vi "Autonomous Independent.vi"   [LabVIEW 2019]
doc: "This VI is called when autonomous begins, and will automatically be terminated when autonomous ends. You can carry out timed or sensor driven robot movement independently without needing to return to the caller."
uses:
  <vilib>/Rock Robotics/WPI/Solenoid/WPI_SolenoidValue.ctl
  <vilib>/Rock Robotics/WPI/ThirdParty/Phoenix-LabVIEW/Motor Controller/Controls/CTRE_Phoenix_MotorControl_ControlMode.ctl
  <vilib>/Rock Robotics/WPI/Utilities/WPI_GetSetVariantRefNum.vi
  <vilib>/Rock Robotics/Network Tables/NT Read String.vi
  <vilib>/Rock Robotics/Network Tables/NT Write Numeric Array.vi
  <vilib>/Rock Robotics/WPI/Solenoid/WPI_SolenoidSetEnum.vi
  <vilib>/addons/control/pid/pid.llb/PID (DBL).vi
  <vilib>/Rock Robotics/Network Tables/NT Read Number.vi
  <vilib>/Rock Robotics/WPI/RobotDrive/WPI_RobotDriveArcadeDrive_Standard(NoSaturation).vi
  <vilib>/Rock Robotics/Network Tables/NT Write Number.vi
  <vilib>/addons/control/pid/NI_PID_pid.lvlib
panel:
  # "Be sure to right-click and choose Data Operations>>Make Current Value default if you want to save the array values with the VI"
types:
  T1 = typedef "WPI_JoystickDevRef.ctl" = cluster{"Device":T2}
  T2 = typedef "WPI_JoystickDeviceEnum.ctl" = enum16{"USB 0", "USB 1", "USB 2", "USB 3", "USB 4", "USB 5"}
  T3 = typedef "WPI_SolenoidValue.ctl" = enum16{"Off", "On", "Forward", "Reverse"}
  T4 = cluster{"proportional gain (Kc)":dbl, "integral time (Ti, min)":dbl, "derivative time (Td, min)":dbl}
  T5 = typedef "WPI_SolenoidDevRef.ctl" = cluster{"DevStatus":errorcluster, "Pneumatics Control Module":u8, "Forward Solenoid Channel":T6, "Reverse Solenoid Channel":T6}
  T6 = typedef "WPI_SolenoidChannel.ctl" = enum8{"Solenoid 0", "Solenoid 1", "Solenoid 2", "Solenoid 3", "Solenoid 4", "Solenoid 5", "Solenoid 6", "Solenoid 7", "Invalid"}
  T7 = typedef "CTRE_Phoenix_MotorControl_ControlMode.ctl" = u16
  T8 = typedef "WPI_SwitchDevRef.ctl" = cluster{"DevStatus":errorcluster, "DIO Channel":T9, "CntIndex":T10, "Normally Closed":bool}
  T9 = typedef "FPGA_DIOChannel.ctl" = enum8{"DIO 0", "DIO 1", "DIO 2", "DIO 3", "DIO 4", "DIO 5", "DIO 6", "DIO 7", "DIO 8", "DIO 9", "DIO MXP 0", "DIO MXP 1", "DIO MXP 2", "DIO MXP 3", "DIO MXP 4", "DIO MXP 5", "DIO MXP 6", "DIO MXP 7", "DIO MXP 8", "DIO MXP 9", "DIO MXP 10", "DIO MXP 11", "DIO MXP 12", "DIO MXP 13", "DIO MXP 14", "DIO MXP 15", "SPI Port CS1", "SPI Port CS2", "SPI Port CS3", "SPI Port MISO", "SPI Port MOSI", "Invalid"}
  T10 = typedef "FPGA_CounterCtrSystemIndex.ctl" = enum8{"Ctr 0", "Ctr 1", "Ctr 2", "Ctr 3", "Ctr 4", "Ctr 5", "Ctr 6", "Ctr 7", "Invalid"}
  T11 = typedef "WPI_MotorControlDeviceRef.ctl" = cluster{"DeviceStatus":errorcluster, "Type":T12, "PWM":cluster{"PWM Channel":T13, "DeadBand":T14}, "CAN":cluster{"Device Number":u8, "SetOutput VI Ref":variant, "GetOutput VI Ref":variant, "Enable VI Ref":variant, "Disable VI Ref":variant, "Data":variant}, "Invert":bool, "DIO PWM":cluster{"PWM \"Enable\" Channel":T13, "DIOChannel":T9, "PWM Rate":dbl}}
  T12 = typedef "WPI_MotorControlType.ctl" = enum16{"PWM", "CAN", "DIO PWM"}
  T13 = typedef "FPGA_DIOPWMChannel.ctl" = enum8{"PWM 0", "PWM 1", "PWM 2", "PWM 3", "PWM 4", "PWM 5", "PWM 6", "PWM 7", "PWM 8", "PWM 9", "PWM MXP 0", "PWM MXP 1", "PWM MXP 2", "PWM MXP 3", "PWM MXP 4", "PWM MXP 5", "PWM MXP 6", "PWM MXP 7", "PWM MXP 8", "PWM MXP 9", "Invalid"}
  T14 = typedef "WPI_PWMDeadband.ctl" = cluster{"Name":string, "maxPositivePwm":i32, "minPositivePwm":i32, "centerPwm":i32, "maxNegativePwm":i32, "minNegativePwm":i32, "angularRange":u16}
  T15 = typedef "WPI_EncoderDevRef.ctl" = cluster{"DevStatus":errorcluster, "EncoderIndex":T16, "CounterIndex":T10, "DistancePerCount":dbl, "Decoding Type":T17}
  T16 = typedef "FPGA_EncoderIdx.ctl" = enum8{"Enc 0", "Enc 1", "Enc 2", "Enc 3", "Enc 4", "Enc 5", "Enc 6", "Enc 7", "Invalid"}
  T17 = typedef "WPI_EncoderType.ctl" = enum16{"1x", "2x", "4x"}
  T18 = typedef "WPI_RobotDriveDevRef.ctl" = cluster{"DevStatus":errorcluster, "Motors[]":T11[], "Square Inputs":bool, "Max Output":dbl}
  T19 = typedef "WPI_DigitalInputDevRef.ctl" = cluster{"DevStatus":errorcluster, "DIO Channel":T9}
diagram:
  (unwired) "This function is run in parallel when the autonomous period begins. It will be terminated automatically when the period ends.\n\nNote that all Driver Station inputs are automatically latched and will not change once auto begins."
  # "The game specific data sent by FMS"
  # "This tells you the autonomous selected in the \ndashboard. Begin.vi publishes the Auto List values\nby writing a constant to the dashboard.\nUpdate the constant to add or modify the name\nof an autonomous."
  # "Every 20ms, report that we are running autonomous\ncode. Loop will abort the same time as the VI."
  # "This gives you the joystick value\nthat is often the throttle"
  # "Use time and/or sensors to control how the robot drives."
  # "This tells you the driver position\nand alliance color"
  n1 = call <vilib>:"WPI_DriverStationGet Alliance Info.vi"() -> ()  [unwired: 12 out]
  n2 = while {
    stop <- FALSE stop-if-true
    n3 = call <vilib>:"WPI_DriverStationReport Robot Code State.vi"("Autonomous"=TRUE) -> ()  [unwired: 10 in, 1 out]
    n4 = Wait (ms)(milliseconds to wait=u32 20) -> ()  [unwired: 1 out]
  }
  n5 = call <vilib>:"WPI_JoystickRefNum Registry Get.vi"("refnum name"="Joystick 0") -> ("JoystickDevRef"=w7:T1)  [unwired: 1 in, 9 out]
  n6 = call <vilib>:"WPI_JoystickGetValues.vi"("JoystickDevRef"=w7) -> ("Axes"=w3:dbl[])  [unwired: 6 in, 4 out]
  n7 = Index Array(array=w3, index=2) -> ()  [unwired: 1 out]
  n8 = call-poly <vilib>:"NT Write Value.vi"("Numeric Array"=w3, "Name"="Joystick 0/Axes") -> ()  [unwired: 9 in, 1 out]
  n9 = call <vilib>:"WPI_DriverStationGame Specific Data.vi"() -> ("Game Specific Data"=w1:string)  [unwired: 11 in]
  n10 = call-poly <vilib>:"NT Read Value.vi"("Name"="Auto Selector") -> ("String"=w4:string)  [unwired: 9 in, 1 out]
  n11 = case shown="\"a\"" w4 {
    tunnel: w1 -> [_ _ _ _ _ _]
    frame Default {
    }
    frame "acc" {
    }
    frame "a" {
      n12 = flat-sequence {
        tunnel: [w67] -> w14
        tunnel: [w66] -> w13
        tunnel: w14 -> [w88]
        tunnel: w13 -> [w89]
        tunnel: [w121] -> w12
        tunnel: w12 -> [w149]
        frame #0 {
          # "turn the light"
          n13 = call <vilib>:"WPI_SolenoidRefNum Registry Get.vi"("refnum name"="led") -> ("error out"=w18:errorcluster, "SolenoidDevRef"=w17:T5)  [unwired: 9 in]
          n14 = call-poly <vilib>:"WPI_SolenoidSet.vi"("error in (no error)"=w18, "Value"=WPI_SolenoidValue."On", "SolenoidDevRef"=w17) -> ()  [unwired: 7 in, 2 out]
        }
        frame #1 {
          w26 = T7 0 items=["PercentOutput"=0, "Position"=1, "Velocity"=2, "Current"=3, "Follower"=5, "MotionProfile"=6, "MotionMagic"=7, "MotionProfileArc"=10, "Disabled"=15] ("Control Mode")
          # "reset all the encoder"
          n15 = while {
            tunnel: [w31] -> w25
            tunnel: [w30] -> w23
            stop <- w30 stop-if-true
            w36 = T7 0 items=["PercentOutput"=0, "Position"=1, "Velocity"=2, "Current"=3, "Follower"=5, "MotionProfile"=6, "MotionMagic"=7, "MotionProfileArc"=10, "Disabled"=15] ("Control Mode")
            n16 = call <vilib>:"WPI_SwitchRefNum Registry Get.vi"("refnum name"="stop") -> ("error out"=w41:errorcluster, "SwitchDevRef"=w40:T8)  [unwired: 9 in]
            n17 = case shown="True" TRUE {
              frame False {
              }
              frame True {
                n18 = call <vilib>:"Zero Yaw.vi"("Zero"=TRUE) -> ()  [unwired: 11 in]
              }
            }
            n19 = call <vilib>:"WPI_SwitchGetLimitValue.vi"("error in (no error)"=w41, "SwitchDevRef"=w40) -> ("Switch Pressed"=w33:bool)  [unwired: 7 in, 2 out]
            n20 = call <vilib>:"CTRE_Phoenix_MotorControl_RefNumRegistryGet.vi"("refnum name"="chain") -> ("error out"=w38:errorcluster, "PhoenixMotorControlDevRef"=w37:T11)  [unwired: 9 in]
            n21 = Equal?(x=w33, y=TRUE) -> (x = y?=w30:bool)
            n22 = call <vilib>:"CTRE_Phoenix_MotorControl_Set.vi"("error in (no error)"=w38, "Output"=-0.8, "Control Mode"=w36, "PhoenixMotorControlDevRef"=w37) -> ("PhoenixMotorControlDevRef"=w31:T11)  [unwired: 6 in, 1 out]
          }
          n23 = call <vilib>:"WPI_EncoderRefNum Registry Get.vi"("refnum name"="angle") -> ("EncoderDevRef"=w19:T15)  [unwired: 9 in, 1 out]
          n24 = call <vilib>:"WPI_EncoderRefNum Registry Get.vi"("refnum name"="move") -> ("EncoderDevRef"=w20:T15)  [unwired: 9 in, 1 out]
          n25 = case shown="True" w23 {
            tunnel: w20 -> [_ w28]
            tunnel: w19 -> [_ w27]
            frame False {
            }
            frame True {
              n26 = call <vilib>:"WPI_EncoderReset.vi"("EncoderDevRef"=w27) -> ()  [unwired: 9 in, 2 out]
              n27 = call <vilib>:"WPI_EncoderReset.vi"("EncoderDevRef"=w28) -> ()  [unwired: 9 in, 2 out]
            }
          }
          n28 = call <vilib>:"CTRE_Phoenix_MotorControl_Set.vi"("Output"=0.0, "Control Mode"=w26, "PhoenixMotorControlDevRef"=w25) -> ()  [unwired: 7 in, 2 out]
        }
        frame #2 {
          w44 = T7 0 items=["PercentOutput"=0, "Position"=1, "Velocity"=2, "Current"=3, "Follower"=5, "MotionProfile"=6, "MotionMagic"=7, "MotionProfileArc"=10, "Disabled"=15] ("Control Mode")
          # "set angle"
          n29 = while {
            tunnel: [w46] -> w45
            stop <- w50 stop-if-true
            w48 = -323.0 ("setpoint")
            w47 = T7 0 items=["PercentOutput"=0, "Position"=1, "Velocity"=2, "Current"=3, "Follower"=5, "MotionProfile"=6, "MotionMagic"=7, "MotionProfileArc"=10, "Disabled"=15] ("Control Mode")
            n30 = call <vilib>:"WPI_EncoderRefNum Registry Get.vi"("refnum name"="angle") -> ("error out"=w57:errorcluster, "EncoderDevRef"=w58:T15)  [unwired: 9 in]
            n31 = call <vilib>:"WPI_EncoderGet.vi"("error in (no error)"=w57, "EncoderDevRef"=w58) -> ("Distance"=w49:dbl)  [unwired: 4 in, 5 out]
            n32 = call-poly <vilib>:"PID.vi"("output range"=cluster{"output high":dbl, "output low":dbl} {"output high"=0.8, "output low"=-0.8}, "PID gains"=T4 {"proportional gain (Kc)"=0.02, "integral time (Ti, min)"=0.0, "derivative time (Td, min)"=0.0}, "process variable"=w49, "setpoint"=w48) -> ("output"=w60:dbl)  [unwired: 6 in, 1 out]
            n33 = call <vilib>:"CTRE_Phoenix_MotorControl_RefNumRegistryGet.vi"("refnum name"="chain") -> ("error out"=w63:errorcluster, "PhoenixMotorControlDevRef"=w64:T11)  [unwired: 9 in]
            n34 = Multiply(x=w60, y=-1.0) -> (x*y=w55:dbl)
            n35 = Add(x=w48, y=-2.0) -> (x+y=w51:dbl)
            n36 = Add(x=w48, y=2.0) -> (x+y=w53:dbl)
            n37 = call <vilib>:"CTRE_Phoenix_MotorControl_Set.vi"("error in (no error)"=w63, "Output"=w55, "Control Mode"=w47, "PhoenixMotorControlDevRef"=w64) -> ("PhoenixMotorControlDevRef"=w46:T11)  [unwired: 6 in, 1 out]
            n38 = In Range and Coerce(upper limit=w53, x=w49, lower limit=w51) -> (In Range?=w50:bool)  [unwired: 1 out]
          }
          n39 = call <vilib>:"CTRE_Phoenix_MotorControl_Set.vi"("Output"=0.0, "Control Mode"=w44, "PhoenixMotorControlDevRef"=w45) -> ()  [unwired: 7 in, 2 out]
        }
        frame #3 {
          # "get the wheel shoot"
          # "preparation"
          n40 = Tick Count (ms)() -> (millisecond timer value=w68:u32)
          n41 = while {
            tunnel: w68 -> [w74]
            tunnel: [w70] -> w66
            tunnel: [w69] -> w67
            stop <- w71 stop-if-true
            w80 = T7 0 items=["PercentOutput"=0, "Position"=1, "Velocity"=2, "Current"=3, "Follower"=5, "MotionProfile"=6, "MotionMagic"=7, "MotionProfileArc"=10, "Disabled"=15] ("Control Mode")
            w84 = T7 0 items=["PercentOutput"=0, "Position"=1, "Velocity"=2, "Current"=3, "Follower"=5, "MotionProfile"=6, "MotionMagic"=7, "MotionProfileArc"=10, "Disabled"=15] ("Control Mode")
            n42 = Tick Count (ms)() -> (millisecond timer value=w75:u32)
            n43 = Subtract(x=w75, y=w74) -> (x-y=w73:u32)
            n44 = call <vilib>:"CTRE_Phoenix_MotorControl_RefNumRegistryGet.vi"("refnum name"="shoot1") -> ("PhoenixMotorControlDevRef"=w78:T11)  [unwired: 9 in, 1 out]
            n45 = Greater Or Equal?(x=w73, y=u32 3000) -> (x >= y?=w71:bool)
            n46 = call <vilib>:"CTRE_Phoenix_MotorControl_RefNumRegistryGet.vi"("refnum name"="shoot2") -> ("error out"=w82:errorcluster, "PhoenixMotorControlDevRef"=w83:T11)  [unwired: 9 in]
            n47 = call <vilib>:"CTRE_Phoenix_MotorControl_Set.vi"("Output"=-1.0, "Control Mode"=w80, "PhoenixMotorControlDevRef"=w78) -> ("PhoenixMotorControlDevRef"=w69:T11)  [unwired: 7 in, 1 out]
            n48 = call <vilib>:"CTRE_Phoenix_MotorControl_Set.vi"("error in (no error)"=w82, "Output"=1.0, "Control Mode"=w84, "PhoenixMotorControlDevRef"=w83) -> ("PhoenixMotorControlDevRef"=w70:T11)  [unwired: 6 in, 1 out]
          }
        }
        frame #4 {
          w87 = T7 0 items=["PercentOutput"=0, "Position"=1, "Velocity"=2, "Current"=3, "Follower"=5, "MotionProfile"=6, "MotionMagic"=7, "MotionProfileArc"=10, "Disabled"=15] ("Control Mode")
          w90 = T7 0 items=["PercentOutput"=0, "Position"=1, "Velocity"=2, "Current"=3, "Follower"=5, "MotionProfile"=6, "MotionMagic"=7, "MotionProfileArc"=10, "Disabled"=15] ("Control Mode")
          # "finish shooting"
          n49 = Tick Count (ms)() -> (millisecond timer value=w93:u32)
          n50 = while {
            tunnel: w93 -> [w111]
            tunnel: w88 -> [w98]
            tunnel: w89 -> [w97]
            tunnel: [w96] -> w91
            tunnel: [w95] -> w85
            tunnel: [w94] -> _
            stop <- w108 stop-if-true
            w103 = T7 0 items=["PercentOutput"=0, "Position"=1, "Velocity"=2, "Current"=3, "Follower"=5, "MotionProfile"=6, "MotionMagic"=7, "MotionProfileArc"=10, "Disabled"=15] ("Control Mode")
            w107 = T7 0 items=["PercentOutput"=0, "Position"=1, "Velocity"=2, "Current"=3, "Follower"=5, "MotionProfile"=6, "MotionMagic"=7, "MotionProfileArc"=10, "Disabled"=15] ("Control Mode")
            w115 = T7 0 items=["PercentOutput"=0, "Position"=1, "Velocity"=2, "Current"=3, "Follower"=5, "MotionProfile"=6, "MotionMagic"=7, "MotionProfileArc"=10, "Disabled"=15] ("Control Mode")
            w116 = T7 0 items=["PercentOutput"=0, "Position"=1, "Velocity"=2, "Current"=3, "Follower"=5, "MotionProfile"=6, "MotionMagic"=7, "MotionProfileArc"=10, "Disabled"=15] ("Control Mode")
            n51 = Tick Count (ms)() -> (millisecond timer value=w112:u32)
            n52 = Subtract(x=w112, y=w111) -> (x-y=w110:u32)
            n53 = call <vilib>:"CTRE_Phoenix_MotorControl_RefNumRegistryGet.vi"("refnum name"="convey2") -> ("PhoenixMotorControlDevRef"=w101:T11)  [unwired: 9 in, 1 out]
            n54 = call <vilib>:"CTRE_Phoenix_MotorControl_RefNumRegistryGet.vi"("refnum name"="convey1") -> ("error out"=w105:errorcluster, "PhoenixMotorControlDevRef"=w106:T11)  [unwired: 9 in]
            n55 = Greater Or Equal?(x=w110, y=u32 3000) -> (x >= y?=w108:bool)
            n56 = call <vilib>:"CTRE_Phoenix_MotorControl_Set.vi"("error in (no error)"=w105, "Output"=0.5, "Control Mode"=w107, "PhoenixMotorControlDevRef"=w106) -> ("PhoenixMotorControlDevRef"=w94:T11)  [unwired: 6 in, 1 out]
            n57 = call <vilib>:"CTRE_Phoenix_MotorControl_Set.vi"("Output"=1.0, "Control Mode"=w116, "PhoenixMotorControlDevRef"=w97) -> ("PhoenixMotorControlDevRef"=w96:T11)  [unwired: 7 in, 1 out]
            n58 = call <vilib>:"CTRE_Phoenix_MotorControl_Set.vi"("Output"=-1.0, "Control Mode"=w115, "PhoenixMotorControlDevRef"=w98) -> ("PhoenixMotorControlDevRef"=w95:T11)  [unwired: 7 in, 1 out]
            n59 = call <vilib>:"CTRE_Phoenix_MotorControl_Set.vi"("Output"=0.5, "Control Mode"=w103, "PhoenixMotorControlDevRef"=w101) -> ()  [unwired: 7 in, 2 out]
          }
          n60 = call <vilib>:"CTRE_Phoenix_MotorControl_Set.vi"("Output"=0.0, "Control Mode"=w90, "PhoenixMotorControlDevRef"=w91) -> ()  [unwired: 7 in, 2 out]
          n61 = call <vilib>:"CTRE_Phoenix_MotorControl_Set.vi"("Output"=0.0, "Control Mode"=w87, "PhoenixMotorControlDevRef"=w85) -> ()  [unwired: 7 in, 2 out]
        }
        frame #5 {
          # "turn the light off"
          n62 = call <vilib>:"WPI_SolenoidRefNum Registry Get.vi"("refnum name"="led") -> ("error out"=w120:errorcluster, "SolenoidDevRef"=w119:T5)  [unwired: 9 in]
          n63 = call-poly <vilib>:"WPI_SolenoidSet.vi"("error in (no error)"=w120, "Value"=WPI_SolenoidValue."Off", "SolenoidDevRef"=w119) -> ()  [unwired: 7 in, 2 out]
        }
        frame #6 {
          # "turn 30 deg"
          n64 = Tick Count (ms)() -> (millisecond timer value=w122:u32)
          n65 = while {
            tunnel: [w129] -> w121
            tunnel: w122 -> [w126]
            stop <- w123 stop-if-true
            n66 = call-poly <vilib>:"NT Read Value.vi"("Name"="/vision/fuseheading") -> ("Numeric"=w142:dbl)  [unwired: 9 in, 1 out]
            n67 = Subtract(x=w142, y=30.0) -> (x-y=w135:dbl)
            n68 = call <vilib>:"WPI_RobotDriveRefNum Registry Get.vi"("refnum name"="Left and Right Motors") -> ("RobotDriveDevRef"=w146:T18)  [unwired: 9 in, 1 out]
            n69 = Less?(x=w135, y=-180.0 ("x-y")) -> (x < y?=w133:bool)
            n70 = Add(x=w135, y=360.0) -> (x+y=w132:dbl)
            n71 = Select(t=w132, s=w133, f=w135) -> (s? t:f=w131:dbl)
            n72 = Greater Or Equal?(x=w135, y=180.0) -> (x >= y?=w140:bool)
            n73 = Subtract(x=w135, y=360.0) -> (x-y=w139:dbl)
            n74 = Select(t=w139, s=w140, f=w131) -> (s? t:f=w128:dbl)
            n75 = Tick Count (ms)() -> (millisecond timer value=w127:u32)
            n76 = Subtract(x=w127, y=w126) -> (x-y=w125:u32)
            n77 = call-poly <vilib>:"PID.vi"("output range"=cluster{"output high":dbl, "output low":dbl} {"output high"=0.6, "output low"=-0.6}, "PID gains"=T4 {"proportional gain (Kc)"=0.13, "integral time (Ti, min)"=0.0, "derivative time (Td, min)"=0.0}, "process variable"=w128, "setpoint"=0.0) -> ("output"=w130:dbl)  [unwired: 6 in, 1 out]
            n78 = Greater Or Equal?(x=w125, y=u32 3000) -> (x >= y?=w123:bool)
            n79 = call-poly <vilib>:"WPI_RobotDriveArcadeDrive.vi"("X axis value"=w130, "RobotDriveDevRef"=w146) -> ("RobotDriveDevRef"=w129:T18)  [unwired: 7 in, 2 out]
          }
        }
        frame #7 {
          n80 = Tick Count (ms)() -> (millisecond timer value=w150:u32)
          n81 = while {
            tunnel: w150 -> [w154]
            tunnel: w149 -> [w152]
            stop <- w153 stop-if-true
            n82 = Tick Count (ms)() -> (millisecond timer value=w155:u32)
            n83 = Subtract(x=w155, y=w154) -> (x-y=w156:u32)
            n84 = Greater Or Equal?(x=w156, y=u32 2000) -> (x >= y?=w153:bool)
            n85 = call-poly <vilib>:"WPI_RobotDriveArcadeDrive.vi"("Y axis value"=0.5, "RobotDriveDevRef"=w152) -> ()  [unwired: 7 in, 3 out]
          }
        }
      }
    }
    frame "b" {
      n86 = flat-sequence {
        tunnel: [w227] -> w174
        tunnel: [w226] -> w173
        tunnel: w174 -> [w250]
        tunnel: w173 -> [w251]
        tunnel: [w249] -> w163
        tunnel: [w248] -> w161
        tunnel: w163 -> [w285]
        tunnel: [w285] -> w162
        tunnel: w161 -> [w284]
        tunnel: [w284] -> w160
        tunnel: [w287] -> w172
        tunnel: [w286] -> w171
        tunnel: [w289] -> w170
        tunnel: w162 -> [w287]
        tunnel: w160 -> [w286]
        tunnel: w172 -> [w327]
        tunnel: w171 -> [w326]
        tunnel: w170 -> [w325]
        tunnel: [w318] -> w169
        tunnel: [w317] -> w168
        tunnel: [w316] -> w167
        tunnel: w169 -> [w386]
        tunnel: [w386] -> w164
        tunnel: w168 -> [w383]
        tunnel: w167 -> [w384]
        tunnel: w164 -> [w400]
        tunnel: [w399] -> w159
        tunnel: w159 -> [w435]
        tunnel: [w435] -> w158
        tunnel: w158 -> [w438]
        tunnel: [w437] -> w166
        tunnel: [w436] -> w165
        tunnel: w166 -> [w475]
        tunnel: w165 -> [w474]
        frame #0 {
          # "turn the light"
          n87 = call <vilib>:"WPI_SolenoidRefNum Registry Get.vi"("refnum name"="led") -> ("error out"=w178:errorcluster, "SolenoidDevRef"=w177:T5)  [unwired: 9 in]
          n88 = call-poly <vilib>:"WPI_SolenoidSet.vi"("error in (no error)"=w178, "Value"=WPI_SolenoidValue."On", "SolenoidDevRef"=w177) -> ()  [unwired: 7 in, 2 out]
        }
        frame #1 {
          w186 = T7 0 items=["PercentOutput"=0, "Position"=1, "Velocity"=2, "Current"=3, "Follower"=5, "MotionProfile"=6, "MotionMagic"=7, "MotionProfileArc"=10, "Disabled"=15] ("Control Mode")
          # "reset all the encoder"
          n89 = while {
            tunnel: [w191] -> w185
            tunnel: [w190] -> w183
            stop <- w190 stop-if-true
            w196 = T7 0 items=["PercentOutput"=0, "Position"=1, "Velocity"=2, "Current"=3, "Follower"=5, "MotionProfile"=6, "MotionMagic"=7, "MotionProfileArc"=10, "Disabled"=15] ("Control Mode")
            n90 = call <vilib>:"WPI_SwitchRefNum Registry Get.vi"("refnum name"="stop") -> ("error out"=w201:errorcluster, "SwitchDevRef"=w200:T8)  [unwired: 9 in]
            n91 = case shown="True" TRUE {
              frame False {
              }
              frame True {
                n92 = call <vilib>:"Zero Yaw.vi"("Zero"=TRUE) -> ()  [unwired: 11 in]
              }
            }
            n93 = call <vilib>:"WPI_SwitchGetLimitValue.vi"("error in (no error)"=w201, "SwitchDevRef"=w200) -> ("Switch Pressed"=w193:bool)  [unwired: 7 in, 2 out]
            n94 = call <vilib>:"CTRE_Phoenix_MotorControl_RefNumRegistryGet.vi"("refnum name"="chain") -> ("error out"=w198:errorcluster, "PhoenixMotorControlDevRef"=w197:T11)  [unwired: 9 in]
            n95 = Equal?(x=w193, y=TRUE) -> (x = y?=w190:bool)
            n96 = call <vilib>:"CTRE_Phoenix_MotorControl_Set.vi"("error in (no error)"=w198, "Output"=-0.8, "Control Mode"=w196, "PhoenixMotorControlDevRef"=w197) -> ("PhoenixMotorControlDevRef"=w191:T11)  [unwired: 6 in, 1 out]
          }
          n97 = call <vilib>:"WPI_EncoderRefNum Registry Get.vi"("refnum name"="angle") -> ("EncoderDevRef"=w179:T15)  [unwired: 9 in, 1 out]
          n98 = call <vilib>:"WPI_EncoderRefNum Registry Get.vi"("refnum name"="move") -> ("EncoderDevRef"=w180:T15)  [unwired: 9 in, 1 out]
          n99 = case shown="True" w183 {
            tunnel: w180 -> [_ w188]
            tunnel: w179 -> [_ w187]
            frame False {
            }
            frame True {
              n100 = call <vilib>:"WPI_EncoderReset.vi"("EncoderDevRef"=w187) -> ()  [unwired: 9 in, 2 out]
              n101 = call <vilib>:"WPI_EncoderReset.vi"("EncoderDevRef"=w188) -> ()  [unwired: 9 in, 2 out]
            }
          }
          n102 = call <vilib>:"CTRE_Phoenix_MotorControl_Set.vi"("Output"=0.0, "Control Mode"=w186, "PhoenixMotorControlDevRef"=w185) -> ()  [unwired: 7 in, 2 out]
        }
        frame #2 {
          w204 = T7 0 items=["PercentOutput"=0, "Position"=1, "Velocity"=2, "Current"=3, "Follower"=5, "MotionProfile"=6, "MotionMagic"=7, "MotionProfileArc"=10, "Disabled"=15] ("Control Mode")
          # "set angle"
          n103 = while {
            tunnel: [w206] -> w205
            stop <- w210 stop-if-true
            w208 = -323.0 ("setpoint")
            w207 = T7 0 items=["PercentOutput"=0, "Position"=1, "Velocity"=2, "Current"=3, "Follower"=5, "MotionProfile"=6, "MotionMagic"=7, "MotionProfileArc"=10, "Disabled"=15] ("Control Mode")
            n104 = call <vilib>:"WPI_EncoderRefNum Registry Get.vi"("refnum name"="angle") -> ("error out"=w217:errorcluster, "EncoderDevRef"=w218:T15)  [unwired: 9 in]
            n105 = call <vilib>:"WPI_EncoderGet.vi"("error in (no error)"=w217, "EncoderDevRef"=w218) -> ("Distance"=w209:dbl)  [unwired: 4 in, 5 out]
            n106 = call-poly <vilib>:"PID.vi"("output range"=cluster{"output high":dbl, "output low":dbl} {"output high"=0.8, "output low"=-0.8}, "PID gains"=T4 {"proportional gain (Kc)"=0.02, "integral time (Ti, min)"=0.0, "derivative time (Td, min)"=0.0}, "process variable"=w209, "setpoint"=w208) -> ("output"=w220:dbl)  [unwired: 6 in, 1 out]
            n107 = call <vilib>:"CTRE_Phoenix_MotorControl_RefNumRegistryGet.vi"("refnum name"="chain") -> ("error out"=w223:errorcluster, "PhoenixMotorControlDevRef"=w224:T11)  [unwired: 9 in]
            n108 = Multiply(x=w220, y=-1.0) -> (x*y=w215:dbl)
            n109 = Add(x=w208, y=-2.0) -> (x+y=w211:dbl)
            n110 = Add(x=w208, y=2.0) -> (x+y=w213:dbl)
            n111 = call <vilib>:"CTRE_Phoenix_MotorControl_Set.vi"("error in (no error)"=w223, "Output"=w215, "Control Mode"=w207, "PhoenixMotorControlDevRef"=w224) -> ("PhoenixMotorControlDevRef"=w206:T11)  [unwired: 6 in, 1 out]
            n112 = In Range and Coerce(upper limit=w213, x=w209, lower limit=w211) -> (In Range?=w210:bool)  [unwired: 1 out]
          }
          n113 = call <vilib>:"CTRE_Phoenix_MotorControl_Set.vi"("Output"=0.0, "Control Mode"=w204, "PhoenixMotorControlDevRef"=w205) -> ()  [unwired: 7 in, 2 out]
        }
        frame #3 {
          # "get the wheel shoot"
          # "preparation"
          n114 = Tick Count (ms)() -> (millisecond timer value=w228:u32)
          n115 = while {
            tunnel: w228 -> [w234]
            tunnel: [w230] -> w226
            tunnel: [w229] -> w227
            stop <- w231 stop-if-true
            w240 = T7 0 items=["PercentOutput"=0, "Position"=1, "Velocity"=2, "Current"=3, "Follower"=5, "MotionProfile"=6, "MotionMagic"=7, "MotionProfileArc"=10, "Disabled"=15] ("Control Mode")
            w244 = T7 0 items=["PercentOutput"=0, "Position"=1, "Velocity"=2, "Current"=3, "Follower"=5, "MotionProfile"=6, "MotionMagic"=7, "MotionProfileArc"=10, "Disabled"=15] ("Control Mode")
            n116 = Tick Count (ms)() -> (millisecond timer value=w235:u32)
            n117 = Subtract(x=w235, y=w234) -> (x-y=w233:u32)
            n118 = call <vilib>:"CTRE_Phoenix_MotorControl_RefNumRegistryGet.vi"("refnum name"="shoot1") -> ("PhoenixMotorControlDevRef"=w238:T11)  [unwired: 9 in, 1 out]
            n119 = Greater Or Equal?(x=w233, y=u32 3000) -> (x >= y?=w231:bool)
            n120 = call <vilib>:"CTRE_Phoenix_MotorControl_RefNumRegistryGet.vi"("refnum name"="shoot2") -> ("error out"=w242:errorcluster, "PhoenixMotorControlDevRef"=w243:T11)  [unwired: 9 in]
            n121 = call <vilib>:"CTRE_Phoenix_MotorControl_Set.vi"("Output"=-1.0, "Control Mode"=w240, "PhoenixMotorControlDevRef"=w238) -> ("PhoenixMotorControlDevRef"=w229:T11)  [unwired: 7 in, 1 out]
            n122 = call <vilib>:"CTRE_Phoenix_MotorControl_Set.vi"("error in (no error)"=w242, "Output"=1.0, "Control Mode"=w244, "PhoenixMotorControlDevRef"=w243) -> ("PhoenixMotorControlDevRef"=w230:T11)  [unwired: 6 in, 1 out]
          }
        }
        frame #4 {
          w247 = T7 0 items=["PercentOutput"=0, "Position"=1, "Velocity"=2, "Current"=3, "Follower"=5, "MotionProfile"=6, "MotionMagic"=7, "MotionProfileArc"=10, "Disabled"=15] ("Control Mode")
          w252 = T7 0 items=["PercentOutput"=0, "Position"=1, "Velocity"=2, "Current"=3, "Follower"=5, "MotionProfile"=6, "MotionMagic"=7, "MotionProfileArc"=10, "Disabled"=15] ("Control Mode")
          # "finish shooting"
          n123 = Tick Count (ms)() -> (millisecond timer value=w255:u32)
          n124 = while {
            tunnel: w255 -> [w274]
            tunnel: w250 -> [w261]
            tunnel: w251 -> [w260]
            tunnel: [w259] -> w253
            tunnel: [w258] -> w245
            tunnel: [w257] -> w248
            tunnel: [w256] -> w249
            stop <- w271 stop-if-true
            w266 = T7 0 items=["PercentOutput"=0, "Position"=1, "Velocity"=2, "Current"=3, "Follower"=5, "MotionProfile"=6, "MotionMagic"=7, "MotionProfileArc"=10, "Disabled"=15] ("Control Mode")
            w270 = T7 0 items=["PercentOutput"=0, "Position"=1, "Velocity"=2, "Current"=3, "Follower"=5, "MotionProfile"=6, "MotionMagic"=7, "MotionProfileArc"=10, "Disabled"=15] ("Control Mode")
            w278 = T7 0 items=["PercentOutput"=0, "Position"=1, "Velocity"=2, "Current"=3, "Follower"=5, "MotionProfile"=6, "MotionMagic"=7, "MotionProfileArc"=10, "Disabled"=15] ("Control Mode")
            w279 = T7 0 items=["PercentOutput"=0, "Position"=1, "Velocity"=2, "Current"=3, "Follower"=5, "MotionProfile"=6, "MotionMagic"=7, "MotionProfileArc"=10, "Disabled"=15] ("Control Mode")
            n125 = Tick Count (ms)() -> (millisecond timer value=w275:u32)
            n126 = Subtract(x=w275, y=w274) -> (x-y=w273:u32)
            n127 = call <vilib>:"CTRE_Phoenix_MotorControl_RefNumRegistryGet.vi"("refnum name"="convey2") -> ("PhoenixMotorControlDevRef"=w264:T11)  [unwired: 9 in, 1 out]
            n128 = call <vilib>:"CTRE_Phoenix_MotorControl_RefNumRegistryGet.vi"("refnum name"="convey1") -> ("error out"=w268:errorcluster, "PhoenixMotorControlDevRef"=w269:T11)  [unwired: 9 in]
            n129 = Greater Or Equal?(x=w273, y=u32 3000) -> (x >= y?=w271:bool)
            n130 = call <vilib>:"CTRE_Phoenix_MotorControl_Set.vi"("error in (no error)"=w268, "Output"=0.5, "Control Mode"=w270, "PhoenixMotorControlDevRef"=w269) -> ("PhoenixMotorControlDevRef"=w256:T11)  [unwired: 6 in, 1 out]
            n131 = call <vilib>:"CTRE_Phoenix_MotorControl_Set.vi"("Output"=1.0, "Control Mode"=w279, "PhoenixMotorControlDevRef"=w260) -> ("PhoenixMotorControlDevRef"=w259:T11)  [unwired: 7 in, 1 out]
            n132 = call <vilib>:"CTRE_Phoenix_MotorControl_Set.vi"("Output"=-1.0, "Control Mode"=w278, "PhoenixMotorControlDevRef"=w261) -> ("PhoenixMotorControlDevRef"=w258:T11)  [unwired: 7 in, 1 out]
            n133 = call <vilib>:"CTRE_Phoenix_MotorControl_Set.vi"("Output"=0.5, "Control Mode"=w266, "PhoenixMotorControlDevRef"=w264) -> ("PhoenixMotorControlDevRef"=w257:T11)  [unwired: 7 in, 1 out]
          }
          n134 = call <vilib>:"CTRE_Phoenix_MotorControl_Set.vi"("Output"=0.0, "Control Mode"=w252, "PhoenixMotorControlDevRef"=w253) -> ()  [unwired: 7 in, 2 out]
          n135 = call <vilib>:"CTRE_Phoenix_MotorControl_Set.vi"("Output"=0.0, "Control Mode"=w247, "PhoenixMotorControlDevRef"=w245) -> ()  [unwired: 7 in, 2 out]
        }
        frame #5 {
          # "turn the light off"
          n136 = call <vilib>:"WPI_SolenoidRefNum Registry Get.vi"("refnum name"="led") -> ("error out"=w283:errorcluster, "SolenoidDevRef"=w282:T5)  [unwired: 9 in]
          n137 = call-poly <vilib>:"WPI_SolenoidSet.vi"("error in (no error)"=w283, "Value"=WPI_SolenoidValue."Off", "SolenoidDevRef"=w282) -> ()  [unwired: 7 in, 2 out]
        }
        frame #6 {
          # "turn 30 deg"
          n138 = Tick Count (ms)() -> (millisecond timer value=w288:u32)
          n139 = while {
            tunnel: [w296] -> w289
            tunnel: w288 -> [w293]
            stop <- w290 stop-if-true
            n140 = call-poly <vilib>:"NT Read Value.vi"("Name"="/vision/fuseheading") -> ("Numeric"=w309:dbl)  [unwired: 9 in, 1 out]
            n141 = Subtract(x=w309, y=30.0) -> (x-y=w302:dbl)
            n142 = call <vilib>:"WPI_RobotDriveRefNum Registry Get.vi"("refnum name"="Left and Right Motors") -> ("RobotDriveDevRef"=w313:T18)  [unwired: 9 in, 1 out]
            n143 = Less?(x=w302, y=-180.0 ("x-y")) -> (x < y?=w300:bool)
            n144 = Add(x=w302, y=360.0) -> (x+y=w299:dbl)
            n145 = Select(t=w299, s=w300, f=w302) -> (s? t:f=w298:dbl)
            n146 = Greater Or Equal?(x=w302, y=180.0) -> (x >= y?=w307:bool)
            n147 = Subtract(x=w302, y=360.0) -> (x-y=w306:dbl)
            n148 = Select(t=w306, s=w307, f=w298) -> (s? t:f=w295:dbl)
            n149 = Tick Count (ms)() -> (millisecond timer value=w294:u32)
            n150 = Subtract(x=w294, y=w293) -> (x-y=w292:u32)
            n151 = call-poly <vilib>:"PID.vi"("output range"=cluster{"output high":dbl, "output low":dbl} {"output high"=0.6, "output low"=-0.6}, "PID gains"=T4 {"proportional gain (Kc)"=0.14, "integral time (Ti, min)"=0.0, "derivative time (Td, min)"=0.0}, "process variable"=w295, "setpoint"=0.0) -> ("output"=w297:dbl)  [unwired: 6 in, 1 out]
            n152 = Greater Or Equal?(x=w292, y=u32 3000) -> (x >= y?=w290:bool)
            n153 = call-poly <vilib>:"WPI_RobotDriveArcadeDrive.vi"("X axis value"=w297, "RobotDriveDevRef"=w313) -> ("RobotDriveDevRef"=w296:T18)  [unwired: 7 in, 2 out]
          }
        }
        frame #7 {
          w324 = T7 0 items=["PercentOutput"=0, "Position"=1, "Velocity"=2, "Current"=3, "Follower"=5, "MotionProfile"=6, "MotionMagic"=7, "MotionProfileArc"=10, "Disabled"=15] ("Control Mode")
          n154 = while {
            tunnel: w327 -> [w367]
            tunnel: w326 -> [w366]
            tunnel: w325 -> [w362]
            tunnel: [w342] -> w322
            tunnel: [w332] -> w321
            tunnel: [w331] -> w318
            tunnel: [w330] -> w317
            tunnel: [w329] -> _
            tunnel: [w329] -> w316
            stop <- w332 stop-if-true
            w361 = T7 0 items=["PercentOutput"=0, "Position"=1, "Velocity"=2, "Current"=3, "Follower"=5, "MotionProfile"=6, "MotionMagic"=7, "MotionProfileArc"=10, "Disabled"=15] ("Control Mode")
            w365 = T7 0 items=["PercentOutput"=0, "Position"=1, "Velocity"=2, "Current"=3, "Follower"=5, "MotionProfile"=6, "MotionMagic"=7, "MotionProfileArc"=10, "Disabled"=15] ("Control Mode")
            w368 = T7 0 items=["PercentOutput"=0, "Position"=1, "Velocity"=2, "Current"=3, "Follower"=5, "MotionProfile"=6, "MotionMagic"=7, "MotionProfileArc"=10, "Disabled"=15] ("Control Mode")
            # "get the balls"
            # "go forward 1480"
            n155 = call <vilib>:"WPI_DigitalInputRefNum Registry Get.vi"("refnum name"="ir1") -> ("DigitalInputDevRef"=w340:T19)  [unwired: 9 in, 1 out]
            n156 = call <vilib>:"WPI_DigitalInputGetValue.vi"("DigitalInputDevRef"=w340) -> ("Value"=w341:bool)  [unwired: 8 in, 2 out]
            n157 = call-poly <vilib>:"NT Read Value.vi"("Name"="/vision/fuseheading") -> ("Numeric"=w356:dbl)  [unwired: 9 in, 1 out]
            n158 = Implies(1:FALSE ("y"), 2:w341) -> (0:w336:bool)
            n159 = Subtract(x=w356, y=30.0) -> (x-y=w349:dbl)
            n160 = Select(t=0.6, s=w336, f=0.0) -> (s? t:f=w333:dbl)
            n161 = Less?(x=w349, y=-180.0 ("x-y")) -> (x < y?=w347:bool)
            n162 = Add(x=w349, y=360.0) -> (x+y=w346:dbl)
            n163 = Select(t=w346, s=w347, f=w349) -> (s? t:f=w345:dbl)
            n164 = Greater Or Equal?(x=w349, y=180.0) -> (x >= y?=w354:bool)
            n165 = Subtract(x=w349, y=360.0) -> (x-y=w353:dbl)
            n166 = call <vilib>:"CTRE_Phoenix_MotorControl_Set.vi"("Output"=w333, "Control Mode"=w361, "PhoenixMotorControlDevRef"=w366) -> ("PhoenixMotorControlDevRef"=w329:T11)  [unwired: 7 in, 1 out]
            n167 = call <vilib>:"CTRE_Phoenix_MotorControl_Set.vi"("Output"=w333, "Control Mode"=w368, "PhoenixMotorControlDevRef"=w367) -> ("PhoenixMotorControlDevRef"=w330:T11)  [unwired: 7 in, 1 out]
            n168 = Select(t=w353, s=w354, f=w345) -> (s? t:f=w344:dbl)
            n169 = call <vilib>:"CTRE_Phoenix_MotorControl_RefNumRegistryGet.vi"("refnum name"="intake") -> ("PhoenixMotorControlDevRef"=w364:T11)  [unwired: 9 in, 1 out]
            n170 = call-poly <vilib>:"PID.vi"("output range"=cluster{"output high":dbl, "output low":dbl} {"output high"=0.5, "output low"=-0.5}, "PID gains"=T4 {"proportional gain (Kc)"=0.13, "integral time (Ti, min)"=0.0, "derivative time (Td, min)"=0.0}, "process variable"=w344, "setpoint"=0.0) -> ("output"=w343:dbl)  [unwired: 6 in, 1 out]
            n171 = call <vilib>:"CTRE_Phoenix_MotorControl_Set.vi"("Output"=-0.7, "Control Mode"=w365, "PhoenixMotorControlDevRef"=w364) -> ("PhoenixMotorControlDevRef"=w342:T11)  [unwired: 7 in, 1 out]
            n172 = call <vilib>:"WPI_EncoderRefNum Registry Get.vi"("refnum name"="move") -> ("EncoderDevRef"=w370:T15)  [unwired: 9 in, 1 out]
            n173 = call <vilib>:"WPI_EncoderGet.vi"("EncoderDevRef"=w370) -> ("Distance"=w373:dbl)  [unwired: 5 in, 5 out]
            n174 = call-poly <vilib>:"PID.vi"("output range"=cluster{"output high":dbl, "output low":dbl} {"output high"=0.5, "output low"=-0.5}, "PID gains"=T4 {"proportional gain (Kc)"=0.02, "integral time (Ti, min)"=0.0, "derivative time (Td, min)"=0.0}, "process variable"=w373, "setpoint"=-1500.0) -> ("output"=w371:dbl)  [unwired: 6 in, 1 out]
            n175 = In Range and Coerce(upper limit=-1480.0, x=w373, lower limit=-1500.0) -> (In Range?=w332:bool)  [unwired: 1 out]
            n176 = call-poly <vilib>:"WPI_RobotDriveArcadeDrive.vi"("Y axis value"=w371, "X axis value"=w343, "RobotDriveDevRef"=w362) -> ("RobotDriveDevRef"=w331:T18)  [unwired: 6 in, 2 out]
          }
          n177 = call <vilib>:"WPI_EncoderRefNum Registry Get.vi"("refnum name"="move") -> ("EncoderDevRef"=w320:T15)  [unwired: 9 in, 1 out]
          n178 = case shown="True" w321 {
            tunnel: w320 -> [_ w328]
            frame False {
            }
            frame True {
              n179 = call <vilib>:"WPI_EncoderReset.vi"("EncoderDevRef"=w328) -> ()  [unwired: 9 in, 2 out]
            }
          }
          n180 = call <vilib>:"CTRE_Phoenix_MotorControl_Set.vi"("Output"=0.0, "Control Mode"=w324, "PhoenixMotorControlDevRef"=w322) -> ()  [unwired: 7 in, 2 out]
        }
        frame #8 {
          w380 = 0.0
          w381 = T7 0 items=["PercentOutput"=0, "Position"=1, "Velocity"=2, "Current"=3, "Follower"=5, "MotionProfile"=6, "MotionMagic"=7, "MotionProfileArc"=10, "Disabled"=15] ("Control Mode")
          w382 = T7 0 items=["PercentOutput"=0, "Position"=1, "Velocity"=2, "Current"=3, "Follower"=5, "MotionProfile"=6, "MotionMagic"=7, "MotionProfileArc"=10, "Disabled"=15] ("Control Mode")
          # "make the balls up in the convey a little bit"
          n181 = Tick Count (ms)() -> (millisecond timer value=w385:u32)
          n182 = while {
            tunnel: w385 -> [w392]
            tunnel: w384 -> [w390]
            tunnel: w383 -> [w389]
            tunnel: [w388] -> w378
            tunnel: [w387] -> w379
            stop <- w391 stop-if-true
            w398 = 0.5
            w397 = T7 0 items=["PercentOutput"=0, "Position"=1, "Velocity"=2, "Current"=3, "Follower"=5, "MotionProfile"=6, "MotionMagic"=7, "MotionProfileArc"=10, "Disabled"=15] ("Control Mode")
            w396 = T7 0 items=["PercentOutput"=0, "Position"=1, "Velocity"=2, "Current"=3, "Follower"=5, "MotionProfile"=6, "MotionMagic"=7, "MotionProfileArc"=10, "Disabled"=15] ("Control Mode")
            # "0.5"
            n183 = Tick Count (ms)() -> (millisecond timer value=w394:u32)
            n184 = Subtract(x=w394, y=w392) -> (x-y=w395:u32)
            n185 = call <vilib>:"CTRE_Phoenix_MotorControl_Set.vi"("Output"=w398, "Control Mode"=w396, "PhoenixMotorControlDevRef"=w390) -> ("PhoenixMotorControlDevRef"=w388:T11)  [unwired: 7 in, 1 out]
            n186 = call <vilib>:"CTRE_Phoenix_MotorControl_Set.vi"("Output"=w398, "Control Mode"=w397, "PhoenixMotorControlDevRef"=w389) -> ("PhoenixMotorControlDevRef"=w387:T11)  [unwired: 7 in, 1 out]
            n187 = Greater Or Equal?(x=w395, y=u32 300) -> (x >= y?=w391:bool)
          }
          n188 = call <vilib>:"CTRE_Phoenix_MotorControl_Set.vi"("Output"=w380, "Control Mode"=w382, "PhoenixMotorControlDevRef"=w378) -> ()  [unwired: 7 in, 2 out]
          n189 = call <vilib>:"CTRE_Phoenix_MotorControl_Set.vi"("Output"=w380, "Control Mode"=w381, "PhoenixMotorControlDevRef"=w379) -> ()  [unwired: 7 in, 2 out]
        }
        frame #9 {
          n190 = while {
            tunnel: w400 -> [w413]
            tunnel: [w411] -> w399
            stop <- w401 stop-if-true
            # "go forward 1480"
            n191 = call-poly <vilib>:"NT Read Value.vi"("Name"="/vision/fuseheading") -> ("Numeric"=w426:dbl)  [unwired: 9 in, 1 out]
            n192 = Subtract(x=w426, y=30.0) -> (x-y=w419:dbl)
            n193 = call <vilib>:"WPI_EncoderRefNum Registry Get.vi"("refnum name"="move") -> ("EncoderDevRef"=w404:T15)  [unwired: 9 in, 1 out]
            n194 = Less?(x=w419, y=-180.0 ("x-y")) -> (x < y?=w417:bool)
            n195 = Add(x=w419, y=360.0) -> (x+y=w416:dbl)
            n196 = call <vilib>:"WPI_EncoderGet.vi"("EncoderDevRef"=w404) -> ("Distance"=w406:dbl)  [unwired: 5 in, 5 out]
            n197 = Select(t=w416, s=w417, f=w419) -> (s? t:f=w415:dbl)
            n198 = call-poly <vilib>:"PID.vi"("output range"=cluster{"output high":dbl, "output low":dbl} {"output high"=0.7, "output low"=-0.7}, "PID gains"=T4 {"proportional gain (Kc)"=0.02, "integral time (Ti, min)"=0.0, "derivative time (Td, min)"=0.0}, "process variable"=w406, "setpoint"=1500.0) -> ("output"=w402:dbl)  [unwired: 6 in, 1 out]
            n199 = Greater Or Equal?(x=w419, y=180.0) -> (x >= y?=w424:bool)
            n200 = Subtract(x=w419, y=360.0) -> (x-y=w423:dbl)
            n201 = In Range and Coerce(upper limit=1500.0, x=w406, lower limit=1480.0) -> (In Range?=w401:bool)  [unwired: 1 out]
            n202 = Select(t=w423, s=w424, f=w415) -> (s? t:f=w414:dbl)
            n203 = call-poly <vilib>:"PID.vi"("output range"=cluster{"output high":dbl, "output low":dbl} {"output high"=0.5, "output low"=-0.5}, "PID gains"=T4 {"proportional gain (Kc)"=0.13, "integral time (Ti, min)"=0.0, "derivative time (Td, min)"=0.0}, "process variable"=w414, "setpoint"=0.0) -> ("output"=w412:dbl)  [unwired: 6 in, 1 out]
            n204 = call-poly <vilib>:"WPI_RobotDriveArcadeDrive.vi"("Y axis value"=w402, "X axis value"=w412, "RobotDriveDevRef"=w413) -> ("RobotDriveDevRef"=w411:T18)  [unwired: 6 in, 2 out]
          }
        }
        frame #10 {
          n205 = call <vilib>:"WPI_SolenoidRefNum Registry Get.vi"("refnum name"="led") -> ("error out"=w434:errorcluster, "SolenoidDevRef"=w433:T5)  [unwired: 9 in]
          n206 = call-poly <vilib>:"WPI_SolenoidSet.vi"("error in (no error)"=w434, "Value"=WPI_SolenoidValue."On", "SolenoidDevRef"=w433) -> ()  [unwired: 7 in, 2 out]
        }
        frame #11 {
          # "turn to 0 deg"
          n207 = Tick Count (ms)() -> (millisecond timer value=w439:u32)
          n208 = while {
            tunnel: [w466] -> w437
            tunnel: [w465] -> w436
            tunnel: w439 -> [w462]
            tunnel: w438 -> [w441]
            stop <- w460 stop-if-true
            w440 = T7 0 items=["PercentOutput"=0, "Position"=1, "Velocity"=2, "Current"=3, "Follower"=5, "MotionProfile"=6, "MotionMagic"=7, "MotionProfileArc"=10, "Disabled"=15] ("Control Mode")
            w473 = T7 0 items=["PercentOutput"=0, "Position"=1, "Velocity"=2, "Current"=3, "Follower"=5, "MotionProfile"=6, "MotionMagic"=7, "MotionProfileArc"=10, "Disabled"=15] ("Control Mode")
            # "-1"
            # "1"
            n209 = call <vilib>:"CTRE_Phoenix_MotorControl_RefNumRegistryGet.vi"("refnum name"="shoot1") -> ("PhoenixMotorControlDevRef"=w469:T11)  [unwired: 9 in, 1 out]
            n210 = call-poly <vilib>:"NT Read Value.vi"("Name"="/vision/fuseheading") -> ("Numeric"=w455:dbl)  [unwired: 9 in, 1 out]
            n211 = call <vilib>:"CTRE_Phoenix_MotorControl_RefNumRegistryGet.vi"("refnum name"="shoot2") -> ("PhoenixMotorControlDevRef"=w472:T11)  [unwired: 9 in, 1 out]
            n212 = call <vilib>:"CTRE_Phoenix_MotorControl_Set.vi"("Output"=-1.0, "Control Mode"=w440, "PhoenixMotorControlDevRef"=w469) -> ("PhoenixMotorControlDevRef"=w466:T11)  [unwired: 7 in, 1 out]
            n213 = call <vilib>:"CTRE_Phoenix_MotorControl_Set.vi"("Output"=1.0, "Control Mode"=w473, "PhoenixMotorControlDevRef"=w472) -> ("PhoenixMotorControlDevRef"=w465:T11)  [unwired: 7 in, 1 out]
            n214 = Subtract(x=w455, y=0.0) -> (x-y=w448:dbl)
            n215 = Add(x=w448, y=360.0) -> (x+y=w445:dbl)
            n216 = Less?(x=w448, y=-180.0 ("x-y")) -> (x < y?=w446:bool)
            n217 = Tick Count (ms)() -> (millisecond timer value=w463:u32)
            n218 = Greater Or Equal?(x=w448, y=180.0) -> (x >= y?=w453:bool)
            n219 = Select(t=w445, s=w446, f=w448) -> (s? t:f=w444:dbl)
            n220 = Subtract(x=w448, y=360.0) -> (x-y=w452:dbl)
            n221 = Subtract(x=w463, y=w462) -> (x-y=w461:u32)
            n222 = Select(t=w452, s=w453, f=w444) -> (s? t:f=w443:dbl)
            n223 = Greater Or Equal?(x=w461, y=u32 3000) -> (x >= y?=w460:bool)
            n224 = call-poly <vilib>:"PID.vi"("output range"=cluster{"output high":dbl, "output low":dbl} {"output high"=0.6, "output low"=-0.6}, "PID gains"=T4 {"proportional gain (Kc)"=0.14, "integral time (Ti, min)"=0.0, "derivative time (Td, min)"=0.0}, "process variable"=w443, "setpoint"=0.0) -> ("output"=w442:dbl)  [unwired: 6 in, 1 out]
            n225 = call-poly <vilib>:"WPI_RobotDriveArcadeDrive.vi"("X axis value"=w442, "RobotDriveDevRef"=w441) -> ()  [unwired: 7 in, 3 out]
          }
        }
        frame #12 {
          w478 = T7 0 items=["PercentOutput"=0, "Position"=1, "Velocity"=2, "Current"=3, "Follower"=5, "MotionProfile"=6, "MotionMagic"=7, "MotionProfileArc"=10, "Disabled"=15] ("Control Mode")
          w480 = T7 0 items=["PercentOutput"=0, "Position"=1, "Velocity"=2, "Current"=3, "Follower"=5, "MotionProfile"=6, "MotionMagic"=7, "MotionProfileArc"=10, "Disabled"=15] ("Control Mode")
          w483 = T7 0 items=["PercentOutput"=0, "Position"=1, "Velocity"=2, "Current"=3, "Follower"=5, "MotionProfile"=6, "MotionMagic"=7, "MotionProfileArc"=10, "Disabled"=15] ("Control Mode")
          w484 = T7 0 items=["PercentOutput"=0, "Position"=1, "Velocity"=2, "Current"=3, "Follower"=5, "MotionProfile"=6, "MotionMagic"=7, "MotionProfileArc"=10, "Disabled"=15] ("Control Mode")
          # "finish shooting"
          # "1"
          # "finish shooting"
          n226 = Tick Count (ms)() -> (millisecond timer value=w488:u32)
          n227 = while {
            tunnel: w488 -> [w507]
            tunnel: w475 -> [w494]
            tunnel: w474 -> [w493]
            tunnel: [w492] -> w486
            tunnel: [w491] -> w476
            tunnel: [w490] -> w477
            tunnel: [w489] -> w479
            stop <- w504 stop-if-true
            w499 = T7 0 items=["PercentOutput"=0, "Position"=1, "Velocity"=2, "Current"=3, "Follower"=5, "MotionProfile"=6, "MotionMagic"=7, "MotionProfileArc"=10, "Disabled"=15] ("Control Mode")
            w503 = T7 0 items=["PercentOutput"=0, "Position"=1, "Velocity"=2, "Current"=3, "Follower"=5, "MotionProfile"=6, "MotionMagic"=7, "MotionProfileArc"=10, "Disabled"=15] ("Control Mode")
            w511 = T7 0 items=["PercentOutput"=0, "Position"=1, "Velocity"=2, "Current"=3, "Follower"=5, "MotionProfile"=6, "MotionMagic"=7, "MotionProfileArc"=10, "Disabled"=15] ("Control Mode")
            w512 = T7 0 items=["PercentOutput"=0, "Position"=1, "Velocity"=2, "Current"=3, "Follower"=5, "MotionProfile"=6, "MotionMagic"=7, "MotionProfileArc"=10, "Disabled"=15] ("Control Mode")
            n228 = Tick Count (ms)() -> (millisecond timer value=w508:u32)
            n229 = Subtract(x=w508, y=w507) -> (x-y=w506:u32)
            n230 = call <vilib>:"CTRE_Phoenix_MotorControl_RefNumRegistryGet.vi"("refnum name"="convey2") -> ("PhoenixMotorControlDevRef"=w497:T11)  [unwired: 9 in, 1 out]
            n231 = call <vilib>:"CTRE_Phoenix_MotorControl_RefNumRegistryGet.vi"("refnum name"="convey1") -> ("error out"=w501:errorcluster, "PhoenixMotorControlDevRef"=w502:T11)  [unwired: 9 in]
            n232 = Greater Or Equal?(x=w506, y=u32 3000) -> (x >= y?=w504:bool)
            n233 = call <vilib>:"CTRE_Phoenix_MotorControl_Set.vi"("error in (no error)"=w501, "Output"=0.5, "Control Mode"=w503, "PhoenixMotorControlDevRef"=w502) -> ("PhoenixMotorControlDevRef"=w489:T11)  [unwired: 6 in, 1 out]
            n234 = call <vilib>:"CTRE_Phoenix_MotorControl_Set.vi"("Output"=1.0, "Control Mode"=w512, "PhoenixMotorControlDevRef"=w493) -> ("PhoenixMotorControlDevRef"=w492:T11)  [unwired: 7 in, 1 out]
            n235 = call <vilib>:"CTRE_Phoenix_MotorControl_Set.vi"("Output"=-1.0, "Control Mode"=w511, "PhoenixMotorControlDevRef"=w494) -> ("PhoenixMotorControlDevRef"=w491:T11)  [unwired: 7 in, 1 out]
            n236 = call <vilib>:"CTRE_Phoenix_MotorControl_Set.vi"("Output"=0.5, "Control Mode"=w499, "PhoenixMotorControlDevRef"=w497) -> ("PhoenixMotorControlDevRef"=w490:T11)  [unwired: 7 in, 1 out]
          }
          n237 = call <vilib>:"CTRE_Phoenix_MotorControl_Set.vi"("Output"=0.0, "Control Mode"=w483, "PhoenixMotorControlDevRef"=w486) -> ()  [unwired: 7 in, 2 out]
          n238 = call <vilib>:"CTRE_Phoenix_MotorControl_Set.vi"("Output"=0.0, "Control Mode"=w484, "PhoenixMotorControlDevRef"=w477) -> ()  [unwired: 7 in, 2 out]
          n239 = call <vilib>:"CTRE_Phoenix_MotorControl_Set.vi"("Output"=0.0, "Control Mode"=w478, "PhoenixMotorControlDevRef"=w476) -> ()  [unwired: 7 in, 2 out]
          n240 = call <vilib>:"CTRE_Phoenix_MotorControl_Set.vi"("Output"=0.0, "Control Mode"=w480, "PhoenixMotorControlDevRef"=w479) -> ()  [unwired: 7 in, 2 out]
        }
        frame #13 {
          n241 = call <vilib>:"WPI_SolenoidRefNum Registry Get.vi"("refnum name"="led") -> ("error out"=w516:errorcluster, "SolenoidDevRef"=w515:T5)  [unwired: 9 in]
          n242 = call-poly <vilib>:"WPI_SolenoidSet.vi"("error in (no error)"=w516, "Value"=WPI_SolenoidValue."Off", "SolenoidDevRef"=w515) -> ()  [unwired: 7 in, 2 out]
        }
      }
    }
    frame "Alternative 1" {
      # "This sample code describes robot movements in an array. You can extend it to control other motors\non your robot. You can also use file I/O to move the data to a text file."
      n243 = while {
        stop <- FALSE stop-if-true
        n244 = call-poly <vilib>:"NT Read Value.vi"("Name"="/vision/balls/x") -> ("Numeric"=w518:dbl)  [unwired: 9 in, 1 out]
        n245 = call-poly <vilib>:"NT Write Value.vi"("Numeric"=w518, "Name"="DB/getBallValue") -> ()  [unwired: 9 in, 1 out]
      }
    }
    frame "Alternative 2" {
      w522 = "RobotDrive Motors" ("Name")
      # "This is some simple sample code to drive your robot curving one direction and then the other."
      # "stand still"
      # "other way for 0.5 second"
      # "turn for 1 second"
      n246 = call <vilib>:"WPI_RobotDriveRefNum Registry Get.vi"("refnum name"="Left and Right Motors") -> ("RobotDriveDevRef"=w538:T18)  [unwired: 1 in, 9 out]
      n247 = call-poly <vilib>:"WPI_RobotDriveArcadeDrive.vi"("Y axis value"=0.5 ("X axis value"), "X axis value"=-0.25, "RobotDriveDevRef"=w538) -> ("Motor Values"=w521:dbl[], "RobotDriveDevRef"=w531:T18)  [unwired: 1 in, 6 out]
      n248 = call <vilib>:"WPI_RobotDriveDelayAndUpdateSafety.vi"("Delay (s)"=1.0, "RobotDriveDevRef"=w531) -> ("RobotDriveDevRef 2"=w532:T18)  [unwired: 8 in, 1 out]
      n249 = call-poly <vilib>:"WPI_RobotDriveArcadeDrive.vi"("Y axis value"=-0.25 ("X axis value"), "X axis value"=0.5, "RobotDriveDevRef"=w532) -> ("Motor Values"=w523:dbl[], "RobotDriveDevRef"=w533:T18)  [unwired: 1 in, 6 out]
      n250 = call <vilib>:"WPI_RobotDriveDelayAndUpdateSafety.vi"("Delay (s)"=0.5, "RobotDriveDevRef"=w533) -> ("RobotDriveDevRef 2"=w534:T18)  [unwired: 8 in, 1 out]
      n251 = call-poly <vilib>:"NT Write Value.vi"("Numeric Array"=w521, "Name"=w522) -> ()  [unwired: 9 in, 1 out]
      n252 = call-poly <vilib>:"NT Write Value.vi"("Numeric Array"=w523, "Name"=w522) -> ()  [unwired: 9 in, 1 out]
      n253 = call-poly <vilib>:"WPI_RobotDriveArcadeDrive.vi"("Y axis value"=0.0 ("X axis value"), "X axis value"=0.0, "RobotDriveDevRef"=w534) -> ("Motor Values"=w524:dbl[])  [unwired: 1 in, 7 out]
      n254 = call-poly <vilib>:"NT Write Value.vi"("Numeric Array"=w524, "Name"=w522) -> ()  [unwired: 9 in, 1 out]
    }
  }
